vi "Teleop.vi"(10 "Match Info":T1={"Autonomous Elapsed Seconds"=0.0, "TeleOp Elapsed Seconds"=0.0, "Disabled Elapsed Seconds"=0.0, "Visited Autonomous"=FALSE, "Visited TeleOp"=FALSE, "Visited Disabled"=FALSE, "Autonomous Settings"={"Autonomous Style"=enum."Independent", "VI Refnum"=refnum}}, 11 "Call Context":T2) -> ()   [LabVIEW 2017]
doc: "This VI is called for each enabled TeleOp packet received from the DS. It is typically used to read from joysticks and other inputs and update I/O or setpoints for timed control loops. It should complete and return within 20 milliseconds or risk missing DS packets."
uses:
  <vilib>/Rock Robotics/WPI/DriverStation/WPI_DriverStationDerivedRobotMode.ctl
  <vilib>/Rock Robotics/WPI/DriverStation/WPI_DriverStationMatch Info.ctl
  <vilib>/Rock Robotics/WPI/Utilities/WPI_GetSetVariantRefNum.vi
  <vilib>/Rock Robotics/Network Tables/NT Write Number.vi
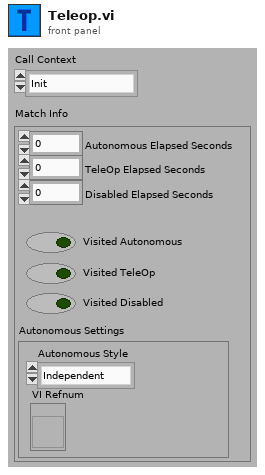
[diagram p1: front panel]
types:
  T1 = typedef "WPI_DriverStationMatch Info.ctl" = cluster{"Autonomous Elapsed Seconds":dbl, "TeleOp Elapsed Seconds":dbl, "Disabled Elapsed Seconds":dbl, "Visited Autonomous":bool, "Visited TeleOp":bool, "Visited Disabled":bool, "Autonomous Settings":cluster{"Autonomous Style":enum16{"Iterative", "Independent"}, "VI Refnum":refnum<vi>}}
  T2 = typedef "WPI_DriverStationDerivedRobotMode.ctl" = enum16{"Init", "Execute", "Stop"}
  T3 = enum16{"Linear", "Square  Root", "Square", "n^x"}
  T4 = typedef "WPI_JoystickDevRef.ctl" = cluster{"Device":T5}
  T5 = typedef "WPI_JoystickDeviceEnum.ctl" = enum16{"USB 0", "USB 1", "USB 2", "USB 3", "USB 4", "USB 5"}
  T6 = cluster{"X":dbl, "Y":dbl, "Angle":dbl, "Magnitude":dbl}
  T7 = typedef "Command Status Info.ctl" = cluster{"Name":string, "Status":T8, "notifier out":T9}
  T8 = typedef "Completion Status.ctl" = enum16{"Successful", "Aborted", "Incomplete"}
  T9 = typedef "Completion Notifier.ctl" = refnum<notifier>
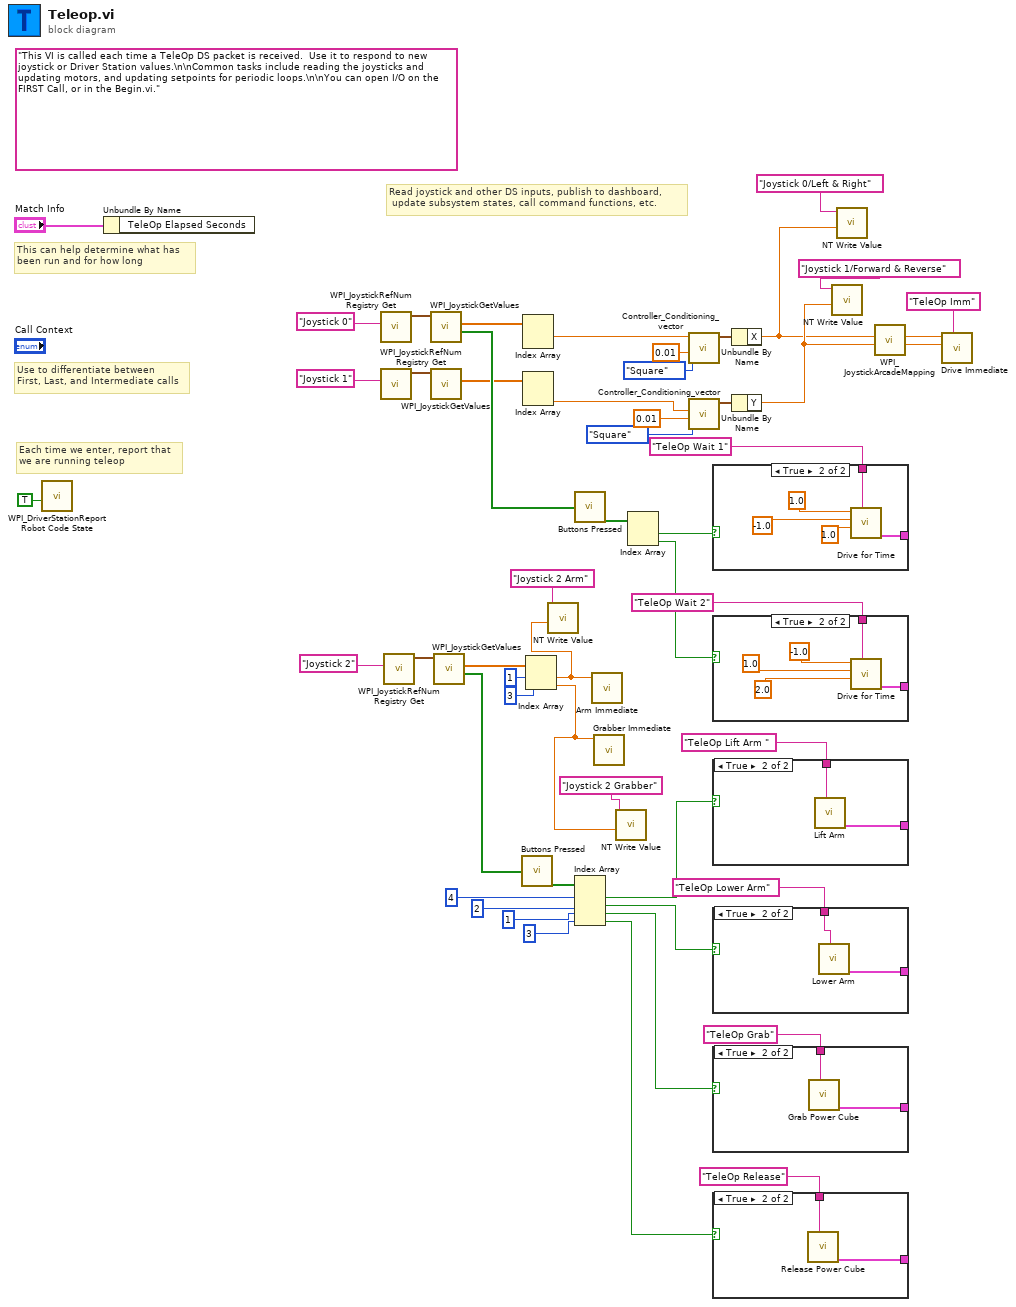
[diagram p0: block diagram]
diagram:
  (unwired) "This VI is called each time a TeleOp DS packet is received.  Use it to respond to new joystick or Driver Station values.\n\nCommon tasks include reading the joysticks and updating motors, and updating setpoints for periodic loops.\n\nYou can open I/O on the FIRST Call, or in the Begin.vi."
  # "Read joystick and other DS inputs, publish to dashboard,\n update subsystem states, call command functions, etc."
  # "Each time we enter, report that\nwe are running teleop"
  # "Use to differentiate between\nFirst, Last, and Intermediate calls"
  # "This can help determine what has\nbeen run and for how long"
  n1 = call <vilib>:"WPI_DriverStationReport Robot Code State.vi"("TeleOp"=TRUE ("Autonomous")) -> ()  [unwired: 10 in, 1 out]
  n2 = Unbundle By Name("Match Info") -> ()  [unwired: 1 out]
  n3 = call <vilib>:"WPI_JoystickRefNum Registry Get.vi"("refnum name"="Joystick 0") -> ("JoystickDevRef"=w49:T4)  [unwired: 1 in, 9 out]
  n4 = call <vilib>:"WPI_JoystickRefNum Registry Get.vi"("refnum name"="Joystick 1") -> ("JoystickDevRef"=w36:T4)  [unwired: 1 in, 9 out]
  n5 = call <vilib>:"WPI_JoystickRefNum Registry Get.vi"("refnum name"="Joystick 2") -> ("JoystickDevRef"=w23:T4)  [unwired: 1 in, 9 out]
  n6 = call <vilib>:"WPI_JoystickGetValues.vi"("JoystickDevRef"=w49) -> ("Buttons"=w40:bool[], "Axes"=w39:dbl[])  [unwired: 6 in, 3 out]
  n7 = call <vilib>:"WPI_JoystickGetValues.vi"("JoystickDevRef"=w36) -> ("Axes"=w38:dbl[])  [unwired: 6 in, 4 out]
  n8 = call <vilib>:"WPI_JoystickGetValues.vi"("JoystickDevRef"=w23) -> ("Buttons"=w13:bool[], "Axes"=w21:dbl[])  [unwired: 6 in, 3 out]
  n9 = call "Buttons Pressed.vi"("Button Values"=w13) -> ("Button Presses"=w14:bool[])
  n10 = Index Array(array=w39) -> (element #1=w33:dbl)  [unwired: 2 in, 1 out]
  n11 = Index Array(array=w38) -> (element #2=w28:dbl)  [unwired: 2 in, 1 out]
  n12 = Index Array(array=w21, index #1=1 ("index"), index #2=3 ("index")) -> (element #1=w16:dbl, element #2=w15:dbl)
  n13 = call-poly <vilib>:"NT Write Value.vi"("Numeric"=w16, "Name"="Joystick 2 Arm") -> ()  [unwired: 9 in, 1 out]
  n14 = call "Buttons Pressed.vi"("Button Values"=w40) -> ("Button Presses"=w45:bool[])
  n15 = Index Array(array=w14, index #1=4 ("index"), index #2=2 ("index"), index #3=1 ("index"), index #4=3 ("index")) -> (element #1=w12:bool, element #2=w11:bool, element #3=w10:bool, element #4=w9:bool)
  n16 = call "Arm Immediate.vi"("Setpoint"=w16) -> ()  [unwired: 10 in, 1 out]
  n17 = call "Grabber Immediate.vi"("Setpoint"=w15) -> ()  [unwired: 10 in, 1 out]
  n18 = call-poly <vilib>:"NT Write Value.vi"("Numeric"=w15, "Name"="Joystick 2 Grabber") -> ()  [unwired: 9 in, 1 out]
  n19 = Index Array(array=w45) -> (element #1=w44:bool, element #2=w43:bool)  [unwired: 2 in]
  n20 = call "Controller_Conditioning_vector.vi"("Enum"=T3."Square", "Dead Zone(0 to 1)"=0.01, "X(-1 to 1)"=w33) -> ("output cluster"=w31:T6)  [unwired: 8 in]
  n21 = call "Controller_Conditioning_vector.vi"("Enum"=T3."Square", "Dead Zone(0 to 1)"=0.01, "Y(-1 to 1)"=w28) -> ("output cluster"=w30:T6)  [unwired: 8 in]
  n22 = case shown="True" w44 {
    tunnel: [_ w56] -> _
    tunnel: "TeleOp Wait 1" ("Description") -> [_ w55]
    frame False {
    }
    frame True {
      n23 = call "Drive for Time.vi"("Description"=w55, "Seconds"=1.0, "Right Speed"=-1.0, "Left Speed"=1.0) -> ("Command Info Out"=w56:T7)  [unwired: 6 in, 1 out]
    }
  }
  n24 = case shown="True" w43 {
    tunnel: [_ w60] -> _
    tunnel: "TeleOp Wait 2" ("Description") -> [_ w59]
    frame False {
    }
    frame True {
      n25 = call "Drive for Time.vi"("Description"=w59, "Seconds"=2.0, "Right Speed"=1.0, "Left Speed"=-1.0) -> ("Command Info Out"=w60:T7)  [unwired: 6 in, 1 out]
    }
  }
  n26 = case shown="True" w12 {
    tunnel: "TeleOp Lift Arm " ("Description") -> [_ w64]
    tunnel: [_ w63] -> _
    frame False {
    }
    frame True {
      n27 = call "Lift Arm.vi"("Description"=w64) -> ("Command Info Out"=w63:T7)  [unwired: 10 in]
    }
  }
  n28 = case shown="True" w11 {
    tunnel: "TeleOp Lower Arm" ("Description") -> [_ w66]
    tunnel: [_ w65] -> _
    frame False {
    }
    frame True {
      n29 = call "Lower Arm.vi"("Description"=w66) -> ("Command Info Out"=w65:T7)  [unwired: 10 in]
    }
  }
  n30 = case shown="True" w10 {
    tunnel: "TeleOp Grab" ("Description") -> [_ w68]
    tunnel: [_ w67] -> _
    frame False {
    }
    frame True {
      n31 = call "Grab Power Cube.vi"("Description"=w68) -> ("Command Info Out"=w67:T7)  [unwired: 10 in]
    }
  }
  n32 = case shown="True" w9 {
    tunnel: "TeleOp Release" ("Description") -> [_ w70]
    tunnel: [_ w69] -> _
    frame False {
    }
    frame True {
      n33 = call "Release Power Cube.vi"("Description"=w70) -> ("Command Info Out"=w69:T7)  [unwired: 10 in]
    }
  }
  n34 = Unbundle By Name(w31) -> ("X"=w26:dbl)
  n35 = Unbundle By Name(w30) -> ("Y"=w27:dbl)
  n36 = call-poly <vilib>:"NT Write Value.vi"("Numeric"=w27, "Name"="Joystick 1/Forward & Reverse") -> ()  [unwired: 9 in, 1 out]
  n37 = call-poly <vilib>:"NT Write Value.vi"("Numeric"=w26, "Name"="Joystick 0/Left & Right") -> ()  [unwired: 9 in, 1 out]
  n38 = call <vilib>:"WPI_JoystickArcadeMapping.vi"("Y axis value"=w27, "X axis value"=w26) -> ("Right Motor Value"=w41:dbl, "Left Motor Value"=w42:dbl)  [unwired: 8 in]
  n39 = call "Drive Immediate.vi"("Description"="TeleOp Imm", "Right Setpoint"=w41, "Left Setpoint"=w42) -> ()  [unwired: 8 in, 1 out]
